vi "Factory (by name).vi"(0 "Obj in":refnum<class "Waveform.lvclass">, 7 "Class Name":string, 11 "error in (no error)":errorcluster) -> (4 "Obj out":refnum<class "Waveform.lvclass">, 15 "error out":errorcluster)   [LabVIEW 2015, in "Waveform.lvclass"]
uses:
  Waveform.lvclass
  Waveform.lvclass/Waveform.ctl
  Tone/Tone.lvclass
  Noise/Noise.lvclass
  Tone Cloud/Tone Cloud.lvclass
  File/File.lvclass
  FM Sweep/FM Sweep.lvclass
  Pulse Train/Pulse Train.lvclass
  Moving Ripple Noise/Moving Ripple Noise.lvclass
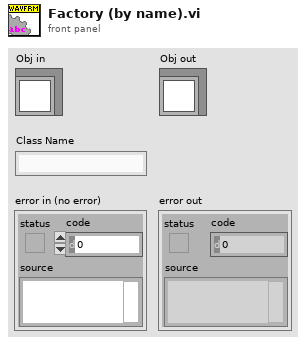
[diagram p1: front panel]
types:
  T1 = typedef "Waveform.lvclass/Serialized.ctl" = cluster{"Numeric":dbl}
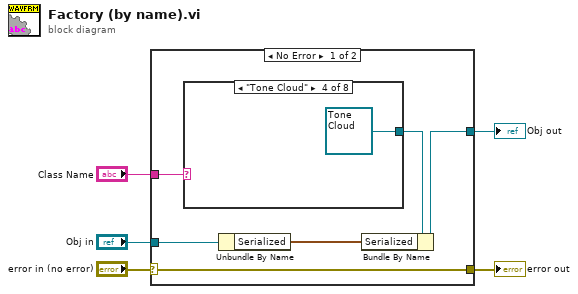
[diagram p0: block diagram]
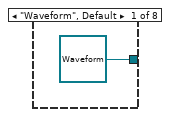
[diagram p2: hidden frame]
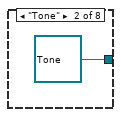
[diagram p3: hidden frame]
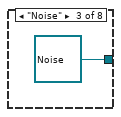
[diagram p4: hidden frame]
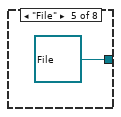
[diagram p5: hidden frame]
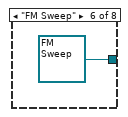
[diagram p6: hidden frame]
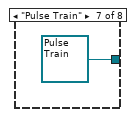
[diagram p7: hidden frame]
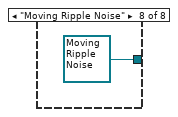
[diagram p8: hidden frame]
diagram:
  n1 = case shown="No Error" "error in (no error)" {
    selector: "error in (no error)" -> [w9 w21]
    tunnel: [w9 w21] -> w4
    tunnel: [w7 w20] -> w2
    tunnel: "Obj in" -> [w8 w20]
    tunnel: "Class Name" -> [w10 _]
    frame No Error {
      n2 = case shown="\"Tone Cloud\"" w10 {
        tunnel: [refnum<class "Waveform.lvclass"> refnum ("Waveform") refnum<class "Tone.lvclass"> refnum ("Tone") refnum<class "Noise.lvclass"> refnum ("Noise") refnum<class "Tone Cloud.lvclass"> refnum ("ToneCloud") refnum<class "File.lvclass"> refnum ("File") refnum<class "FM Sweep.lvclass"> refnum ("FM Sweep") refnum<class "Pulse Train.lvclass"> refnum ("Pulse Train") refnum<class "Moving Ripple Noise.lvclass"> refnum ("Moving Ripple Noise")] -> w11
        frame "Waveform", Default {
        }
        frame "Tone" {
        }
        frame "Noise" {
        }
        frame "Tone Cloud" {
        }
        frame "File" {
        }
        frame "FM Sweep" {
        }
        frame "Pulse Train" {
        }
        frame "Moving Ripple Noise" {
        }
      }
      n3 = Unbundle By Name(w8) -> ("Serialized"=w6:T1)
      n4 = Bundle By Name(cluster=w11, "Serialized"=w6) -> (w7:refnum<class "Waveform.lvclass">)
    }
    frame Error {
    }
  }
  "error out" <- w4
  "Obj out" <- w2
